vi "Read (Multiple Digital Waveforms).vi"(8 "error in (no error)":errorcluster, 9 "Maximum Time (10000ms)":u32=10000, 10 "Digital Channels":u16[](array[ring])=[14] items=["Digital Channel D0"=14, "Digital Channel D1"=15, "Digital Channel D2"=16, "Digital Channel D3"=17, "Digital Channel D4"=18, "Digital Channel D5"=19, "Digital Channel D6"=20, "Digital Channel D7"=21, "Digital Channel D8"=22, "Digital Channel D9"=23, "Digital Channel D10"=24, "Digital Channel D11"=25, "Digital Channel D12"=26, "Digital Channel D13"=27, "Digital Channel D14"=28, "Digital Channel D15"=29], 11 "VISA resource name":refnum<visa-resource-name>) -> (0 "error out":errorcluster, 2 "Digital Waveform Graph":digitalwaveform[](graph), 3 "VISA resource name out":refnum<visa-resource-name>)   [LabVIEW 2017, in "Scope.lvlib" / "Tektronix DPO MSO 2000 4000 Series.lvlib"]
doc: "Initiates an acquisition on all channels that you enabled with the <B>Configure Digital Channel</B> VI. The VI waits for the acquisition to complete and returns the waveform for the <B>Digital Channels</B> you specified. The <B>Maximum Time</B> control specifies the maximum time to wait for operation complete in milliseconds. If the oscilloscope did not complete the acquisition within the time period you specify with the <B>Maximum Time</B> parameter, the VI returns a timeout error. A common cause for a timeout error is the acquisition was not triggered. For example, the trigger level is out of range of the waveform. \n\n<B>Note:</B> LabVIEW versions higher than 7.1 might display the data differently."
uses:
  Tektronix DPO MSO 2000 4000 Series.lvlib
  Data_Low Level/Fetch Waveform (Digital Waveform).vi
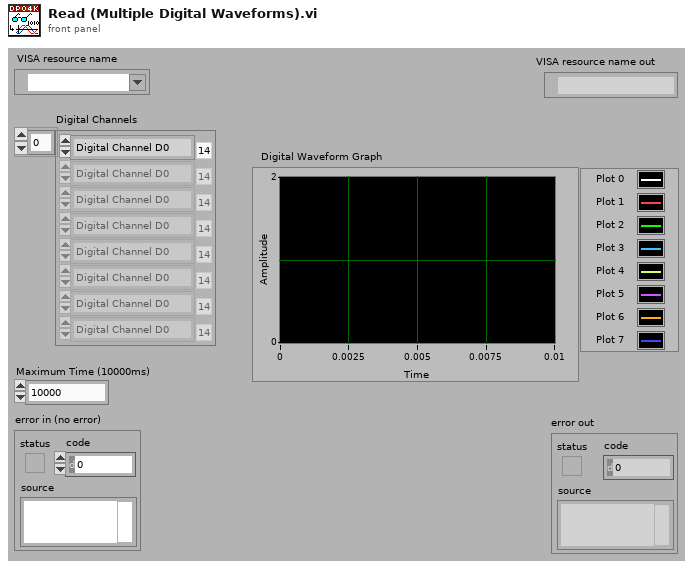
[diagram p1: front panel]
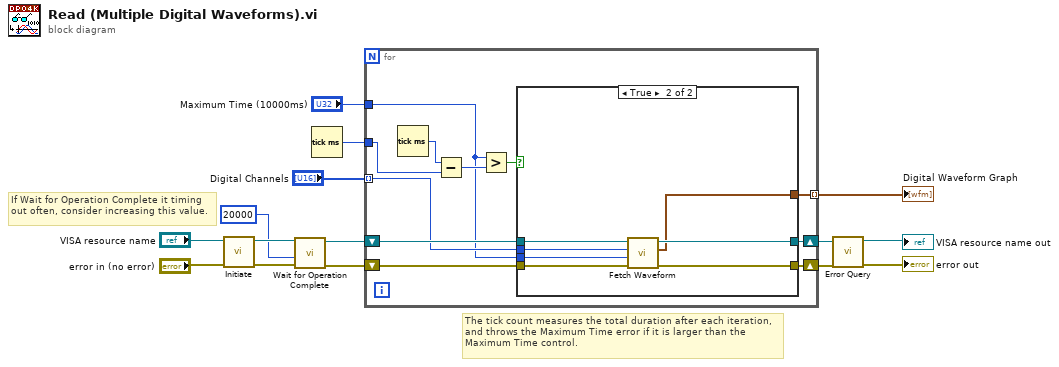
[diagram p0: block diagram]
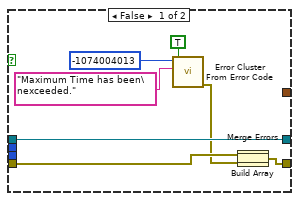
[diagram p2: hidden frame]
diagram:
  # "If Wait for Operation Complete it timing out often, consider increasing this value."
  # "The tick count measures the total duration after each iteration, and throws the Maximum Time error if it is larger than the Maximum Time control."
  n1 = call "Initiate.vi"("error in (no error)"="error in (no error)", "VISA resource name"="VISA resource name") -> ("error out"=w7:errorcluster, "VISA resource name out"=w8:refnum<visa-resource-name>)  [unwired: 8 in]
  n2 = call "Wait for Operation Complete.vi"("error in (no error)"=w7, "Maximum Time (10000ms)"=u32 20000, "VISA resource name"=w8) -> ("error out"=w5:errorcluster, "VISA resource name out"=w6:refnum<visa-resource-name>)  [unwired: 7 in]
  n3 = Tick Count (ms)() -> (millisecond timer value=w3:u32)
  n4 = for {
    shift-right: [w24] -> w14
    shift-left: w6 -> [w25]
    shift-right: [w23] -> w13
    shift-left: w5 -> [w26]
    tunnel: "Digital Channels" -> [w22] mode=indexing
    tunnel: w3 -> [w20]
    tunnel: "Maximum Time (10000ms)" -> [w16]
    tunnel: [w17] -> w1 mode=indexing
    n5 = Tick Count (ms)() -> (millisecond timer value=w21:u32)
    n6 = Subtract(x=w21, y=w20) -> (x-y=w19:u32)
    n7 = Greater?(x=w16, y=w19) -> (0:w18:bool)
    n8 = case shown="True" w18 {
      tunnel: w26 -> [w29 w41]
      tunnel: w25 -> [w34 w40]
      tunnel: [w34 w39] -> w24
      tunnel: [w30 w38] -> w23
      tunnel: w22 -> [_ w37]
      tunnel: [_ w36] -> w17
      tunnel: w16 -> [_ w35]
      frame False {
        n9 = call <vilib>:"Error Cluster From Error Code.vi"("show call chain? (False)"=TRUE, "error message (\"\")"="Maximum Time has been\nexceeded." ("error message (\"\")"), "error code (0)"=-1074004013) -> ("error out"=w28:errorcluster)  [unwired: 6 in]
        n10 = Build Array(w29, w28) -> (w27:errorcluster[])
        n11 = Merge Errors(w27) -> (w30:errorcluster)
      }
      frame True {
        n12 = call-poly "Fetch Waveform.vi"("error in (no error)"=w41, "Maximum Time (10000 ms)"=w35, "Digital Channel (14: Digital Channel D0)"=w37, "VISA resource name"=w40) -> ("error out"=w38:errorcluster, "Digital Waveform"=w36:digitalwaveform, "VISA resource name out"=w39:refnum<visa-resource-name>)  [unwired: 5 in]
      }
    }
  }
  "Digital Waveform Graph" <- w1
  n13 = call "Error Query.vi"("error in (no error)"=w13, "VISA resource name"=w14) -> ("error out"=→"error out":errorcluster, "VISA resource name out"=→"VISA resource name out":refnum<visa-resource-name>)  [unwired: 6 in, 2 out]
